vi "comm unlock2.vi"(8 "error in (no error)":errorcluster, 9 "Locked?":bool=TRUE, 11 "Comm Handle":u32) -> (0 "error out":errorcluster, 3 "dup Comm Handle":u32)   [LabVIEW 2013, in "lvserial.lvlib"]
doc: "Unlocks the serial port."
uses:
  lvserial.lvlib
  lvserial.dll
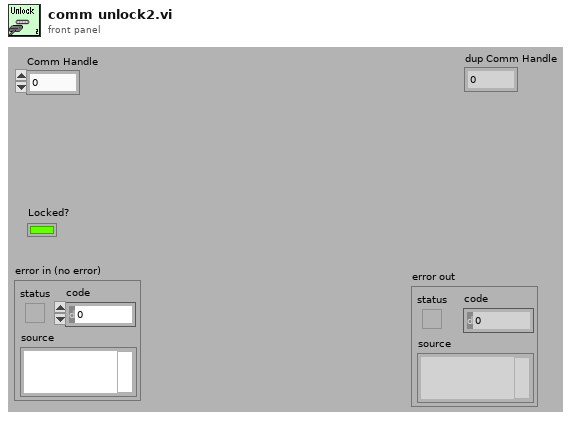
[diagram p1: front panel]
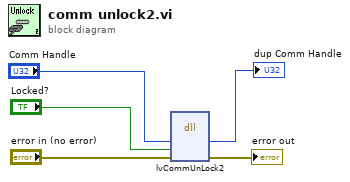
[diagram p0: block diagram]
diagram:
  n1 = dll-call lib="lvserial.dll" fn="lvCommUnLock2"("hComm"="Comm Handle", "Locked?"="Locked?", "error in (no error)"="error in (no error)") -> ("hComm"=→"dup Comm Handle":u32, "error in (no error)"=→"error out":errorcluster)  [unwired: 4 in, 3 out]
